vi "InitialiseChannelsAngle.vi"(0 "Number of data bits":i32, 5 "Fs":dbl, 11 "error in":errorcluster) -> (4 "output cluster":T1, 15 "error out":errorcluster)   [LabVIEW 2021]
uses:
  <vilib>/DAQmx/create/channels.llb/DAQmx Create Channel (DI-Digital Input).vi
  <vilib>/DAQmx/configure/timing.llb/DAQmx Timing (Sample Clock).vi
  <vilib>/DAQmx/create/channels.llb/DAQmx Create Channel (CO-Pulse Generation-Time).vi
  <vilib>/DAQmx/create/channels.llb/DAQmx Create Channel (CO-Pulse Generation-Frequency).vi
  <vilib>/DAQmx/configure/timing.llb/DAQmx Timing (Implicit).vi
  <vilib>/DAQmx/configure/trigger.llb/DAQmx Start Trigger (Digital Edge).vi
  <resource>/objmgr/daqmx.rc
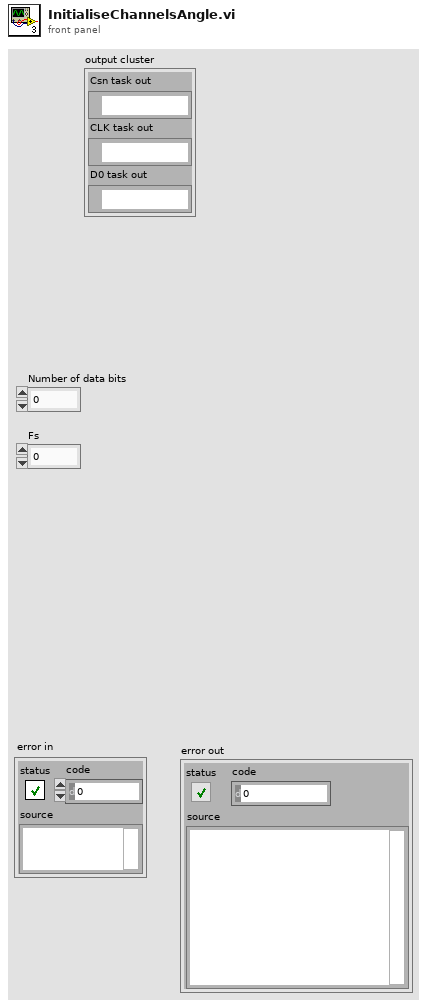
[diagram p1: front panel]
types:
  T1 = cluster{"Csn task out":refnum<k21>, "CLK task out":refnum<k21>, "D0 task out":refnum<k21>}
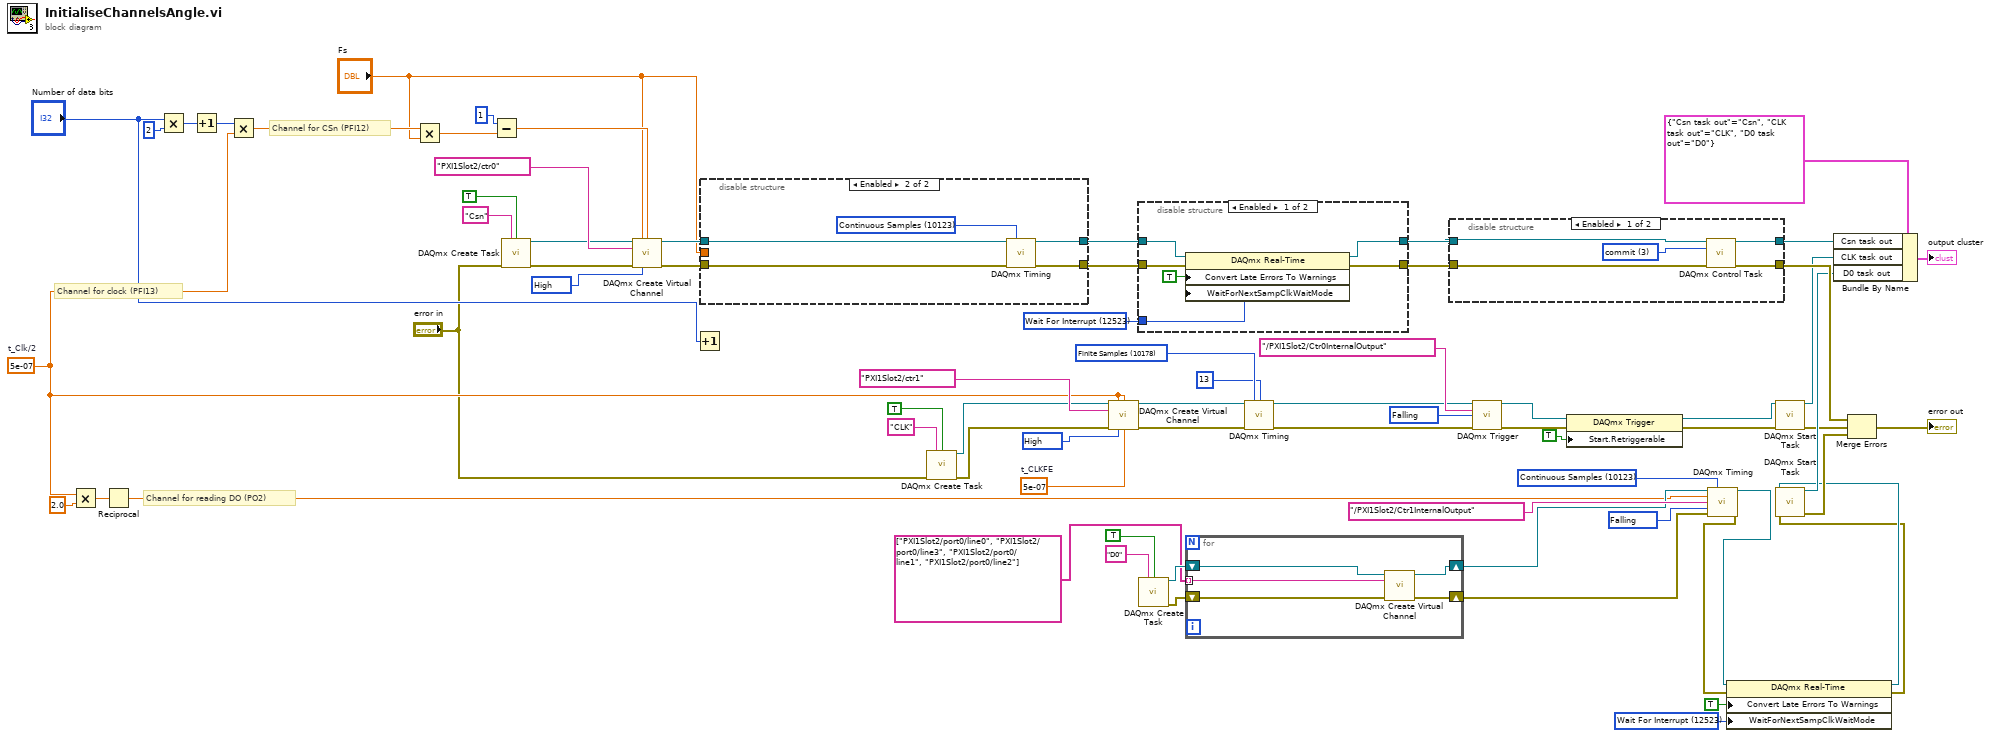
[diagram p0: block diagram]
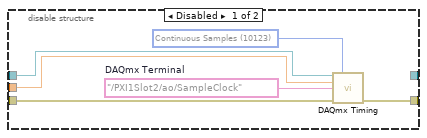
[diagram p3: hidden frame]
diagram:
  w4 = 12523 items=["Wait For Interrupt"=12523, "Poll"=12524] ("WaitForNextSampClkWaitMode")
  w8 = 12523 items=["Wait For Interrupt"=12523, "Poll"=12524] ("WaitForNextSampClkWaitMode")
  w66 = 10192 items=["High"=10192, "Low"=10214] ("idle state")
  w65 = 5e-07  # t_CLKFE
  w56 = 10171 items=["Rising"=10280, "Falling"=10171] ("edge")
  w50 = 10178 items=["Finite Samples"=10178, "Continuous Samples"=10123, "Hardware Timed Single Point"=12522] ("sample mode")
  w48 = 10192 items=["High"=10192, "Low"=10214] ("idle state")
  w26 = 5e-07  # t_Clk/2
  w43 = 10171 items=["Rising"=10280, "Falling"=10171] ("active edge")
  w42 = 10123 items=["Finite Samples"=10178, "Continuous Samples"=10123, "Hardware Timed Single Point"=12522] ("sample mode")
  # "Channel for clock (PFI13)"
  # "Channel for CSn (PFI12)"
  # "Channel for reading DO (PO2)"
  n1 = Multiply(x=w26, y=2.0) -> (x*y=w63:dbl)
  n2 = Reciprocal(x=w63) -> (1/x=w25:dbl)
  n3 = Multiply(x="Number of data bits", y=2) -> (x*y=w45:i32)
  n4 = Increment(x=w45) -> (x+1=w46:i32)
  n5 = Multiply(x=w46, y=w26) -> (x*y=w47:dbl)
  n6 = Multiply(x=w47, y="Fs") -> (x*y=w70:dbl)
  n7 = Subtract(x=1, y=w70) -> (x-y=w69:dbl)
  n8 = call <vilib>:"DAQmx Create Task.vi"("new task name"="Csn", "auto cleanup"=TRUE, "error in"="error in") -> ("task out"=w24:refnum<k21>, "error out"=w34:errorcluster)  [unwired: 11 in]
  n9 = call-poly <vilib>:"DAQmx Create Virtual Channel.vi"("task in"=w24, "frequency"="Fs", "duty cycle"=w69, "counter"=tag "PXI1Slot2/ctr0", "error in"=w34, "idle state"=w66) -> ("task out"=w61:refnum<k21>, "error out"=w62:errorcluster)  [unwired: 8 in]
  n10 = Increment(x="Number of data bits") -> ()  [unwired: 1 out]
  n11 = disable-structure shown="Enabled" {
    disable-tunnel: [w79 w84] -> w10
    disable-tunnel: w62 -> [w78 w83]
    disable-tunnel: w61 -> [w77 w82]
    disable-tunnel: "Fs" -> [w73 _]
    disable-tunnel: [_ w80] -> w12
    frame Disabled {
      w74 = tag "/PXI1Slot2/ao/SampleClock"  # DAQmx Terminal
      w75 = 10123 items=["Finite Samples"=10178, "Continuous Samples"=10123, "Hardware Timed Single Point"=12522] ("sample mode")
      n12 = call-poly <vilib>:"DAQmx Timing.vi"("task/channels in"=w77, "sample mode"=w75, "rate"=w73, "source"=w74, "error in"=w78) -> ("task out"=w76:refnum<k21>, "error out"=w79:errorcluster)  [unwired: 9 in]
    }
    frame Enabled {
      w81 = 10123 items=["Finite Samples"=10178, "Continuous Samples"=10123, "Hardware Timed Single Point"=12522] ("sample mode")
      n13 = call-poly <vilib>:"DAQmx Timing.vi"("task/channels in"=w82, "sample mode"=w81, "error in"=w83) -> ("task out"=w80:refnum<k21>, "error out"=w84:errorcluster)  [unwired: 11 in]
    }
  }
  n14 = call <vilib>:"DAQmx Create Task.vi"("new task name"="CLK", "auto cleanup"=TRUE, "error in"="error in") -> ("task out"=w30:refnum<k21>, "error out"=w31:errorcluster)  [unwired: 11 in]
  n15 = call-poly <vilib>:"DAQmx Create Virtual Channel.vi"("task in"=w30, "high time"=w26, "low time"=w26, "counter"=tag "PXI1Slot2/ctr1", "error in"=w31, "idle state"=w48, "initial delay"=w65) -> ("task out"=w51:refnum<k21>, "error out"=w52:errorcluster)  [unwired: 7 in]
  n16 = disable-structure shown="Enabled" {
    disable-tunnel: w12 -> [w90 w92]
    disable-tunnel: [w89 w92] -> w11
    disable-tunnel: w10 -> [w88 w91]
    disable-tunnel: [w87 w91] -> w9
    disable-tunnel: w8 -> [w85 _]
    frame Enabled {
      n17 = property class="DAQmx Real-Time"(reference=w90, error in=w88, "Convert Late Errors To Warnings"=TRUE ("ConvLateErrorsToWarnings"), "WaitForNextSampClkWaitMode"=w85) -> (reference out=w89:refnum<k21>, error out=w87:errorcluster)
    }
    frame Disabled {
    }
  }
  n18 = call <vilib>:"DAQmx Create Task.vi"("new task name"="D0", "auto cleanup"=TRUE) -> ("task out"=w41:refnum<k21>, "error out"=w40:errorcluster)  [unwired: 12 in]
  n19 = for {
    tunnel: tag[] ["PXI1Slot2/port0/line0", "PXI1Slot2/port0/line3", "PXI1Slot2/port0/line1", "PXI1Slot2/port0/line2"] ("DAQmx Output Channels") -> [w95] mode=indexing
    shift-right: [w94] -> w38
    shift-left: w41 -> [w97]
    shift-right: [w93] -> w37
    shift-left: w40 -> [w96]
    n20 = call-poly <vilib>:"DAQmx Create Virtual Channel.vi"("task in"=w97, "lines"=w95, "error in"=w96) -> ("task out"=w94:refnum<k21>, "error out"=w93:errorcluster)  [unwired: 11 in]
  }
  n21 = call-poly <vilib>:"DAQmx Timing.vi"("task/channels in"=w51, "sample mode"=w50, "samples per channel"=13, "error in"=w52) -> ("task out"=w53:refnum<k21>, "error out"=w54:errorcluster)  [unwired: 10 in]
  n22 = disable-structure shown="Enabled" {
    disable-tunnel: [w102 w103] -> w35
    disable-tunnel: w11 -> [w100 w104]
    disable-tunnel: w9 -> [w99 w103]
    disable-tunnel: [w98 w104] -> w22
    frame Enabled {
      w101 = 3 items=["verify"=2, "reserve"=4, "commit"=3, "unreserve"=5, "abort"=6] ("action")
      n23 = call <vilib>:"DAQmx Control Task.vi"("task/channels in"=w100, "action"=w101, "error in"=w99) -> ("task out"=w98:refnum<k21>, "error out"=w102:errorcluster)  [unwired: 11 in]
    }
    frame Disabled {
    }
  }
  n24 = call-poly <vilib>:"DAQmx Trigger.vi"("task/channels in"=w53, "source"=tag "/PXI1Slot2/Ctr0InternalOutput", "edge"=w56, "error in"=w54) -> ("task out"=w57:refnum<k21>, "error out"=w59:errorcluster)  [unwired: 10 in]
  n25 = property class="DAQmx Trigger"(reference=w57, error in=w59, "Start.Retriggerable"=TRUE) -> (reference out=w21:refnum<k21>, error out=w17:errorcluster)
  n26 = call-poly <vilib>:"DAQmx Timing.vi"("task/channels in"=w38, "sample mode"=w42, "rate"=w25, "source"=tag "/PXI1Slot2/Ctr1InternalOutput", "active edge"=w43, "error in"=w37) -> ("task out"=w6:refnum<k21>, "error out"=w2:errorcluster)  [unwired: 8 in]
  n27 = property class="DAQmx Real-Time"(reference=w6, error in=w2, "Convert Late Errors To Warnings"=TRUE ("ConvLateErrorsToWarnings"), "WaitForNextSampClkWaitMode"=w4) -> (reference out=w5:refnum<k21>, error out=w1:errorcluster)
  n28 = call <vilib>:"DAQmx Start Task.vi"("task/channels in"=w21, "error in"=w17) -> ("task out"=w20:refnum<k21>, "error out"=w18:errorcluster)  [unwired: 12 in]
  n29 = call <vilib>:"DAQmx Start Task.vi"("task/channels in"=w5, "error in"=w1) -> ("task out"=w19:refnum<k21>, "error out"=w16:errorcluster)  [unwired: 12 in]
  n30 = Bundle By Name(cluster=T1 {"Csn task out"="Csn", "CLK task out"="CLK", "D0 task out"="D0"}, "Csn task out"=w22, "CLK task out"=w20, "D0 task out"=w19) -> (→"output cluster":T1)
  n31 = Merge Errors(w35, w18, w16) -> (→"error out":errorcluster)
